vi "Query Elog State.vi"(8 "error in":errorcluster, 11 "VISA resource name":refnum<visa-resource-name>) -> (0 "error out":errorcluster, 2 "State":string, 3 "VISA resource name out":refnum<visa-resource-name>)   [LabVIEW 2024, in "IT-M3900C.lvlib"]
doc: "This command is used to query the ELOG status."
uses:
  IT-M3900C.lvlib
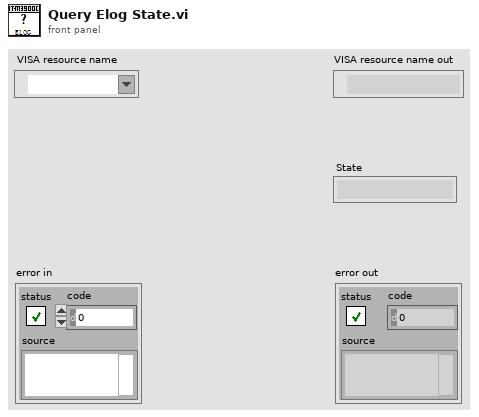
[diagram p1: front panel]
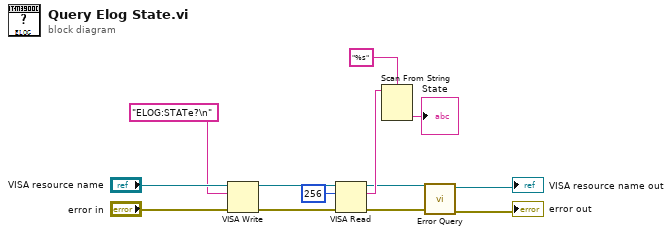
[diagram p0: block diagram]
diagram:
  n1 = VISA Write(VISA resource name="VISA resource name", write buffer="ELOG:STATe?\n" ("写入缓冲区"), error in (no error)="error in") -> (VISA resource name out=w10:refnum<visa-resource-name>, error out=w9:errorcluster)  [unwired: 1 out]
  n2 = VISA Read(VISA resource name=w10, byte count=u32 256 ("字节总数"), error in (no error)=w9) -> (VISA resource name out=w5:refnum<visa-resource-name>, read buffer=w6:string, error out=w4:errorcluster)  [unwired: 1 out]
  n3 = Scan From String(format string="%s" ("格式字符串"), input string=w6) -> (output 1=→"State":string)  [unwired: 3 in, 3 out]
  n4 = call "Error Query.vi"("error in"=w4, "VISA resource name"=w5) -> ("error out"=→"error out":errorcluster, "VISA resource name out"=→"VISA resource name out":refnum<visa-resource-name>)  [unwired: 6 in, 2 out]
